vi "Upload to Sift.vi"(0 "API GRPC URL":string, 1 "Absolute Filepath":path, 5 "API Key":string, 7 "error in (no error)":errorcluster, 9 "Asset Name":string="LabVIEW-TDMS-Example", 11 "Run Name":string="TDMS Upload Example", 12 "API REST URL":string) -> (4 "Run URL":string, 15 "Error":errorcluster)   [LabVIEW 2024, in "Sift TDMS Uploader.lvlib" / "Sift TDMS Uploader.lvclass"]
doc: "Uploads TDMS file to Sift with provided Run and Asset"
uses:
  Sift TDMS Uploader.lvclass
  Sift TDMS Uploader.lvclass/Sift TDMS Uploader.ctl
  <vilib>/Sift/Sift/Sift API/Sift Client.lvclass
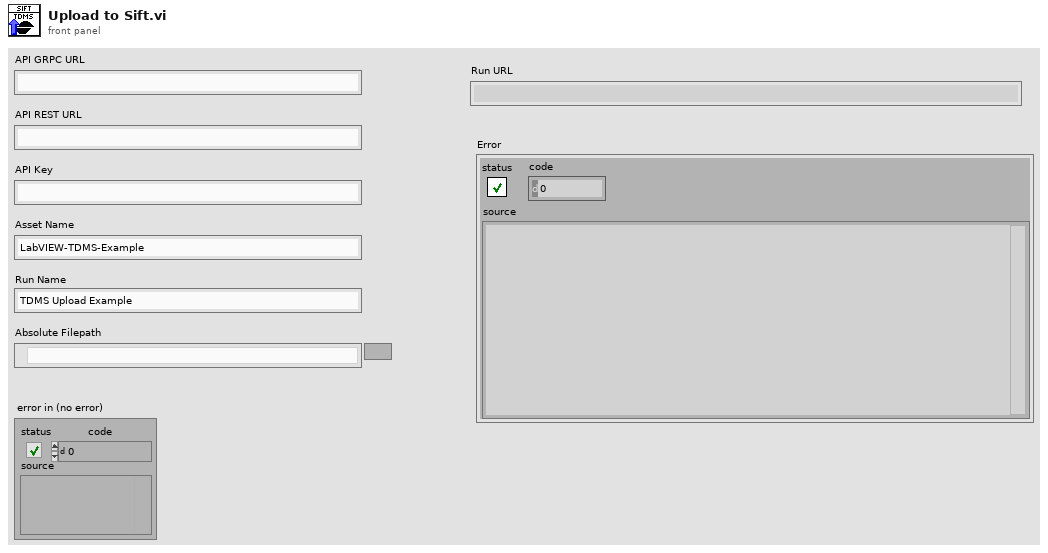
[diagram p1: front panel]
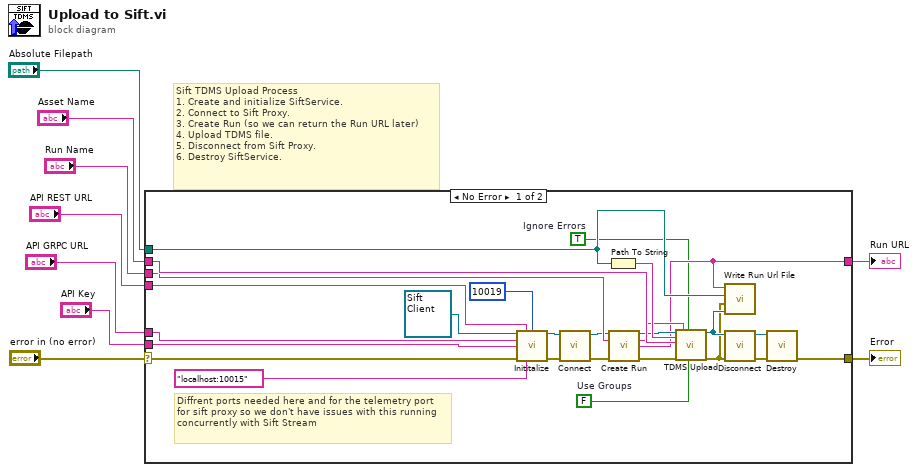
[diagram p0: block diagram]
diagram:
  # "Sift TDMS Upload Process\n1. Create and initialize SiftService.\n2. Connect to Sift Proxy.\n3. Create Run (so we can return the Run URL later)\n4. Upload TDMS file.\n5. Disconnect from Sift Proxy.\n6. Destroy SiftService."
  n1 = case shown="No Error" "error in (no error)" {
    selector: "error in (no error)" -> [w14 w36]
    tunnel: [w34 w36] -> w9
    tunnel: "Asset Name" -> [w30 _]
    tunnel: "API GRPC URL" -> [w27 _]
    tunnel: "API Key" -> [w26 _]
    tunnel: "API REST URL" -> [w25 _]
    tunnel: "Run Name" -> [w24 _]
    tunnel: "Absolute Filepath" -> [w18 _]
    tunnel: [w17 _] -> w2
    frame No Error {
      w11 = TRUE  # Ignore Errors
      w12 = FALSE  # Use Groups
      # "Diffrent ports needed here and for the telemetry port for sift proxy so we don't have issues with this running concurrently with Sift Stream"
      n2 = call-dynamic "Inititalize.vi"("Sift Client in"=refnum<class "Sift Client.lvclass"> refnum ("Sift Client.lvlib:Sift Client.lvclass"), "REST URL"=w25, "Telemetry Port"=u16 10019, "GRPC URL"=w27, "API Key"=w26, "error in (no error)"=w14, "Sift Proxy Address"="localhost:10015") -> ("Sift Client out"=w33:refnum<class "Sift Client.lvclass">, "error out"=w28:errorcluster)  [unwired: 7 in]
      n3 = call-dynamic "Connect.vi"("error in (no error)"=w28, "Sift Client in"=w33) -> ("error out"=w23:errorcluster, "Sift Client out"=w20:refnum<class "Sift Client.lvclass">)  [unwired: 7 in, 1 out]
      n4 = Path To String(path=w18) -> (string=w29:string)
      n5 = call-dynamic "Create Run.vi"("Sift Client in"=w20, "Name"=w24, "error in (no error)"=w23) -> ("Sift Client out"=w19:refnum<class "Sift Client.lvclass">, "Run ID"=w21:string, "URL"=w17:string, "error out"=w22:errorcluster)  [unwired: 9 in]
      n6 = call-dynamic "TDMS Upload.vi"("Sift Client in"=w19, "Filepath"=w29, "Asset Name"=w30, "error in (no error)"=w22, "Run ID"=w21, "Ignore Errors"=w11, "Group Into Components"=w12) -> ("Sift Client out"=w16:refnum<class "Sift Client.lvclass">, "error out"=w15:errorcluster)  [unwired: 11 in]
      n7 = call "Write Run Url File.vi"("Sift Client in"=w16, "error in (no error)"=w15, "TDMS Filepath"=w18, "Run URL"=w17) -> ()  [unwired: 8 in]
      n8 = call-dynamic "Disconnect.vi"("error in (no error)"=w15, "Sift Client in"=w16) -> ("error out"=w31:errorcluster, "Sift Client out"=w32:refnum<class "Sift Client.lvclass">)  [unwired: 8 in]
      n9 = call-dynamic "Destroy.vi"("error in (no error)"=w31, "Sift Client in"=w32) -> ("error out"=w34:errorcluster)  [unwired: 8 in, 1 out]
    }
    frame Error {
    }
  }
  "Error" <- w9
  "Run URL" <- w2
